vi "Server_01.vi"() -> ()   [LabVIEW 2010]
doc: "Demonstrates how to set up a basic TCP connection, send data to the specified port once a connection has been established, and terminate the connection once the data has been sent. This VI is designed to stop if the TCP connection is terminated.\n\nThe data sent in this example is an array consisting of one of three user selectable waveforms.\n\n<B>Note:</B> Requires the Simple Data Client.vi located in the same library as this VI."
uses:
  <vilib>/Analysis/NI_AALBase.lvlib
panel:
  in  "stop":bool
  in  "# of Points":i32=200
  in  "Function":u16(ring) items=["Random", "Sine wave", "Chirp Pattern"]
  in  "Port":u16=2055 min=1025 step=1
  # "Instructions:\n1. Open the Simple Data Client.vi.\n2. Run this VI first.\n3. Run the Simple Data Client.vi second.\n4. Adjust the Function and # of Points controls to see the plot on the front panel of the Simple Data Client.vi change.\n\nNote:  This VI will time out after 60 seconds if no connection is detected."
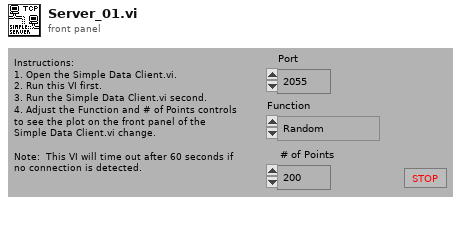
[diagram p1: front panel]
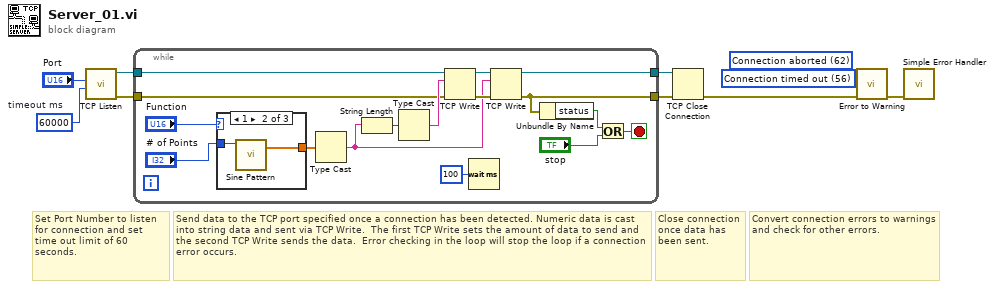
[diagram p0: block diagram]
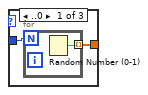
[diagram p2: hidden frame]
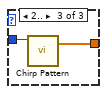
[diagram p3: hidden frame]
diagram:
  w1 = 60000  # timeout ms
  w6 = 56 items=["No Error", "Argument Error", "Memory Full", "Out of Zone", "End of File", "File Already Open", "Generic File IO Error", "File Not Found", "File Permission Error", "Disk Full", "Duplicate Path", "Too Many Files Open", "Not Enabled", "Resource File Not Found", "Cannot Add Resource", "Resource Not Found", "Image Not Found", "Image Memory Error", "Pen Does Not Exist", "Config Bad Type", "Config Token Not Found", "Config Parse Error", "Config Memory Error", "Bad External Code Format", "Bad External Code Offset", "External Code Not Present", "Null Window", "Destroy Window Mixup", "Null Menu", "Print Aborted", "Bad Print Record", "Print Driver Error", "Windows Error During Print", "Memory Error During Print", "Print Dialog Error", "Generic Print Error", "Invalid Device Refnum", "Device Not Found", "Device Parameter Error", "Device Unit Error", "Can't Open Device", "Device Call Aborted", "Generic Error", "Cancelled By User", "Object ID Too Low", "Object ID Too High", "Object Not In Heap", "Unknown Heap", "Bad DefProc ID", "DefProc Not In Table", "Message Out Of Range", "Null Method", "Unknown Message", "Manager Call Not Supported", "Bad address", "Connection In progress", "Connection timed out", "Connection is already in progress", "Network attribute not supported", "Network error", "Address in use", "System out of memory", "Connection aborted", "Connection refused", "Connection is not connected", "Connection is already connected", "Connection closed", "Initialize error (interapplication manager)", "Bad occurrence", "Wait on unbound occurrence handler", "Occurrence queue overflow", "Bad path", "Semaphore not signaled", "Unrecognized type (interapplication manager)"] ("2nd Error to Convert")
  w7 = 62 items=["No Error", "Argument Error", "Memory Full", "Out of Zone", "End of File", "File Already Open", "Generic File IO Error", "File Not Found", "File Permission Error", "Disk Full", "Duplicate Path", "Too Many Files Open", "Not Enabled", "Resource File Not Found", "Cannot Add Resource", "Resource Not Found", "Image Not Found", "Image Memory Error", "Pen Does Not Exist", "Config Bad Type", "Config Token Not Found", "Config Parse Error", "Config Memory Error", "Bad External Code Format", "Bad External Code Offset", "External Code Not Present", "Null Window", "Destroy Window Mixup", "Null Menu", "Print Aborted", "Bad Print Record", "Print Driver Error", "Windows Error During Print", "Memory Error During Print", "Print Dialog Error", "Generic Print Error", "Invalid Device Refnum", "Device Not Found", "Device Parameter Error", "Device Unit Error", "Can't Open Device", "Device Call Aborted", "Generic Error", "Cancelled By User", "Object ID Too Low", "Object ID Too High", "Object Not In Heap", "Unknown Heap", "Bad DefProc ID", "DefProc Not In Table", "Message Out Of Range", "Null Method", "Unknown Message", "Manager Call Not Supported", "Bad address", "Connection In progress", "Connection timed out", "Connection is already in progress", "Network attribute not supported", "Network error", "Address in use", "System out of memory", "Connection aborted", "Connection refused", "Connection is not connected", "Connection is already connected", "Connection closed", "Initialize error (interapplication manager)", "Bad occurrence", "Wait on unbound occurrence handler", "Occurrence queue overflow", "Bad path", "Semaphore not signaled", "Unrecognized type (interapplication manager)"] ("1st Error to Convert")
  # "Convert connection errors to warnings and check for other errors."
  # "Close connection once data has been sent."
  # "Send data to the TCP port specified once a connection has been detected. Numeric data is cast into string data and sent via TCP Write.  The first TCP Write sets the amount of data to send and the second TCP Write sends the data.  Error checking in the loop will stop the loop if a connection error occurs."
  # "Set Port Number to listen for connection and set time out limit of 60 seconds."
  n1 = call <vilib>:"TCP Listen.vi"("timeout ms (wait forever: -1)"=w1, "port"="Port") -> ("error out"=w2:errorcluster, "connection ID"=w4:refnum<k5>)  [unwired: 6 in, 2 out]
  n2 = while {
    tunnel: [w17] -> w3
    tunnel: [w26] -> w5
    tunnel: w4 -> [w25]
    tunnel: w2 -> [w12]
    stop <- w16 stop-if-true
    n3 = case shown="1" "Function" {
      tunnel: "# of Points" -> [w28 w31 w33]
      tunnel: [w27 w30 w32] -> w14
      frame ..0 {
        n4 = for {
          N: w28 -> [_]
          tunnel: [w29] -> w27 mode=indexing
          n5 = Random Number (0-1)() -> (number: 0 to 1=w29:dbl)
        }
      }
      frame 1 {
        n6 = call <vilib>:"Sine Pattern.vi"("samples"=w31) -> ("Sinusoidal Pattern"=w30:dbl[])  [unwired: 3 in, 1 out]
      }
      frame 2.. {
        n7 = call <vilib>:"Chirp Pattern.vi"("samples"=w33) -> ("Chirp Pattern"=w32:dbl[])  [unwired: 3 in, 1 out]
      }
    }
    n8 = Type Cast(x=w14) -> (*(type *) &x=w19:string)  [unwired: 1 in]
    n9 = String Length(string=w19) -> (length=w22:i32)
    n10 = Type Cast(x=w22) -> (*(type *) &x=w21:string)  [unwired: 1 in]
    n11 = TCP Write(connection ID=w25, data in=w21, error in (no error)=w12) -> (connection ID out=w24:refnum<k5>, error out=w23:errorcluster)  [unwired: 1 in, 1 out]
    n12 = Wait (ms)(milliseconds to wait=u32 100) -> ()  [unwired: 1 out]
    n13 = TCP Write(connection ID=w24, data in=w19, error in (no error)=w23) -> (connection ID out=w26:refnum<k5>, error out=w17:errorcluster)  [unwired: 1 in, 1 out]
    n14 = Unbundle By Name(w17) -> ("status"=w15:bool)
    n15 = Or(x=w15, y="stop") -> (x .or. y?=w16:bool)
  }
  n16 = TCP Close Connection(connection ID=w5, error in (no error)=w3) -> (error out=w9:errorcluster)  [unwired: 1 in, 1 out]
  n17 = call <vilib>:"Error to Warning.vi"("1st Error to Convert"=w7, "2nd Error to Convert"=w6, "error in"=w9) -> ("warning out"=w8:errorcluster)  [unwired: 12 in]
  n18 = call <vilib>:"Simple Error Handler.vi"("error in (no error)"=w8) -> ()  [unwired: 4 in, 5 out]
